vi "坐标旋转.vi"   [LabVIEW 2012, in "几何工具.lvlib"]
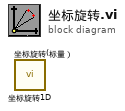
[diagram p0: block diagram]
diagram:
  n1 = call "坐标旋转1D.vi"() -> ()  [unwired: 10 in, 2 out]
  n2 = call "坐标旋转(标量）.vi"() -> ()  [unwired: 10 in, 2 out]
